vi "PID_2Chan_V4_1loop_multiTs_globals.vi"() -> ()   [LabVIEW 2016]
uses:
  <vilib>/addons/control/pid/pid.llb/PID Advanced (DBL Array).vi
  <vilib>/addons/control/pid/pid.llb/PID Parameter Manager (DBL Array).vi
  <vilib>/addons/control/pid/pid.llb/PID Derivative Action Buffered (DBL Array).vi
  <vilib>/addons/control/pid/pid.llb/PID Get Advanced Error (DBL Array).vi
  <vilib>/addons/control/pid/pid.llb/PID Integral Action Buffered (DBL Array).vi
  <vilib>/addons/control/pid/pid.llb/PID Resize 1D Array.vi
  <vilib>/addons/control/pid/pid.llb/PID Get Advanced Error (DBL).vi
  <userlib>/Fluigent/Fluigent MFCS/FluigentMFCS_Full.llb/MFCS_EZ Detect.vi
  <userlib>/Fluigent/Fluigent MFCS/FluigentMFCS_Full.llb/MFCS_EZ Initialization.vi
  <userlib>/Fluigent/Fluigent MFCS/FluigentMFCS_Full.llb/MFCS_EZ Write Channel Pressure.vi
  Globals/PressuresGlobal.vi
  <userlib>/Fluigent/Fluigent MFCS/FluigentMFCS_Full.llb/MFCS_EZ Close.vi
  <vilib>/addons/control/pid/NI_PID_pid.lvlib
  <vilib>/Analysis/NI_AALBase.lvlib
  <vilib>/Analysis/baseanly.llb/Mean (DBL).vi
panel:
  in  "Odor Mix Pressure":dbl
  in  "Set Ctr/Set Odor Mix":bool
  in  "Odor Mix Flowboard":enum16{"A", "B", "C"}(ring)
  in  "Water Mix Flowboard":enum16{"A", "B", "C"}(ring)
  in  "Ctr Water Flowboard":enum16{"A", "B", "C"}(ring)
  in  "Ctr Water":enum16{"1", "2", "3", "4", "5", "6", "7", "8"}(ring)=enum."7"
  in  "Odor Mix":enum16{"1", "2", "3", "4", "5", "6", "7", "8"}(ring)
  in  "Water Mix":enum16{"1", "2", "3", "4", "5", "6", "7", "8"}(ring)=enum."5"
  in  "Total Odor Flow":dbl=425.0
  in  "Ftot Setpoint":dbl=531.25
  in  "AutoControl PID":bool
  out "Pressure Stable?":bool=TRUE
  in  "Ftot Stability Threshold 2":dbl=0.631165
  in  "F1 Stability Threshold":dbl=0.631165
  out "Setpoint Reached?":bool
  in  "Pressure Resolution":dbl=0.631165
  in  "Control Pressure":dbl=270.0 format="%_6g"
  in  "Control Pressure Channel":i16=1
  in  "output cluster":T1
  out "Set Pressure":dbl[](array[numeric])=[924.5131355020292, 768.8474129854441] format="%_10g"
  in  "linearity":dbl[](array[numeric])=[0.30000000000000004, 0.4] format="%.2f"
  out "Flow 1 plot 2":cluster{"[0]":dbl, "[1]":dbl}(graph)={"[0]"=531.25, "[1]"=683.6630748754509}
  out "Flow Rates":dbl[](array[numeric])=[-432.47356854362795, 683.6630748754509]
  in  "FTot PID gains":cluster{"P":dbl, "I":dbl, "D":dbl}={"P"=0.02, "I"=0.0, "D"=0.0} {"D" format="%.3f"; "I" format="%.3f"; "P" format="%.5f"}
  in  "Vals to display":dbl=1235.0
  out "Flow 1 plot":cluster{"[0]":dbl, "[1]":dbl}(graph)={"[0]"=-432.47356854362795, "[1]"=225.0}
  out "Ferr":T2(graph)={"output[0]"=0.5012669198666482, "output[1]"=-3.4973900073056177, "output[2]"=0.0}
  out "Pressures":dbl[](array[numeric])=[901.3263549804688, 1487.6934814453125]
  in  "F1 PID gains":cluster{"P":dbl, "I":dbl, "D":dbl}={"P"=0.004, "I"=0.0, "D"=0.0} {"D" format="%.3f"; "I" format="%.3f"; "P" format="%.5f"}
  in  "reset Averging":bool
  in  "Set current Pressure\n to manual pressure":bool=TRUE
  out "Pressures":T3(graph)={"[0]"=901.3263549804688, "[1]"=1487.6934814453125, "[2]"=924.5131355020292, "[3]"=768.8474129854441}
  in  "stop":bool=TRUE
  in  "Control Valves":enum16{"1", "2", "3", "4", "5", "6", "7", "8"}[](array[ring])=[enum."7"]
  in  "Pressure Channels":i16[](array[numeric])=[2, 3]
  in  "reinitialize? (F)":bool
  in  "Add Ctrl?":bool
  in  "Boards":enum16{"A", "B", "C"}[](array[ring])=[enum."A", enum."A"]
  in  "Valves":enum16{"1", "2", "3", "4", "5", "6", "7", "8"}[](array[ring])=[enum."5", enum."1"]
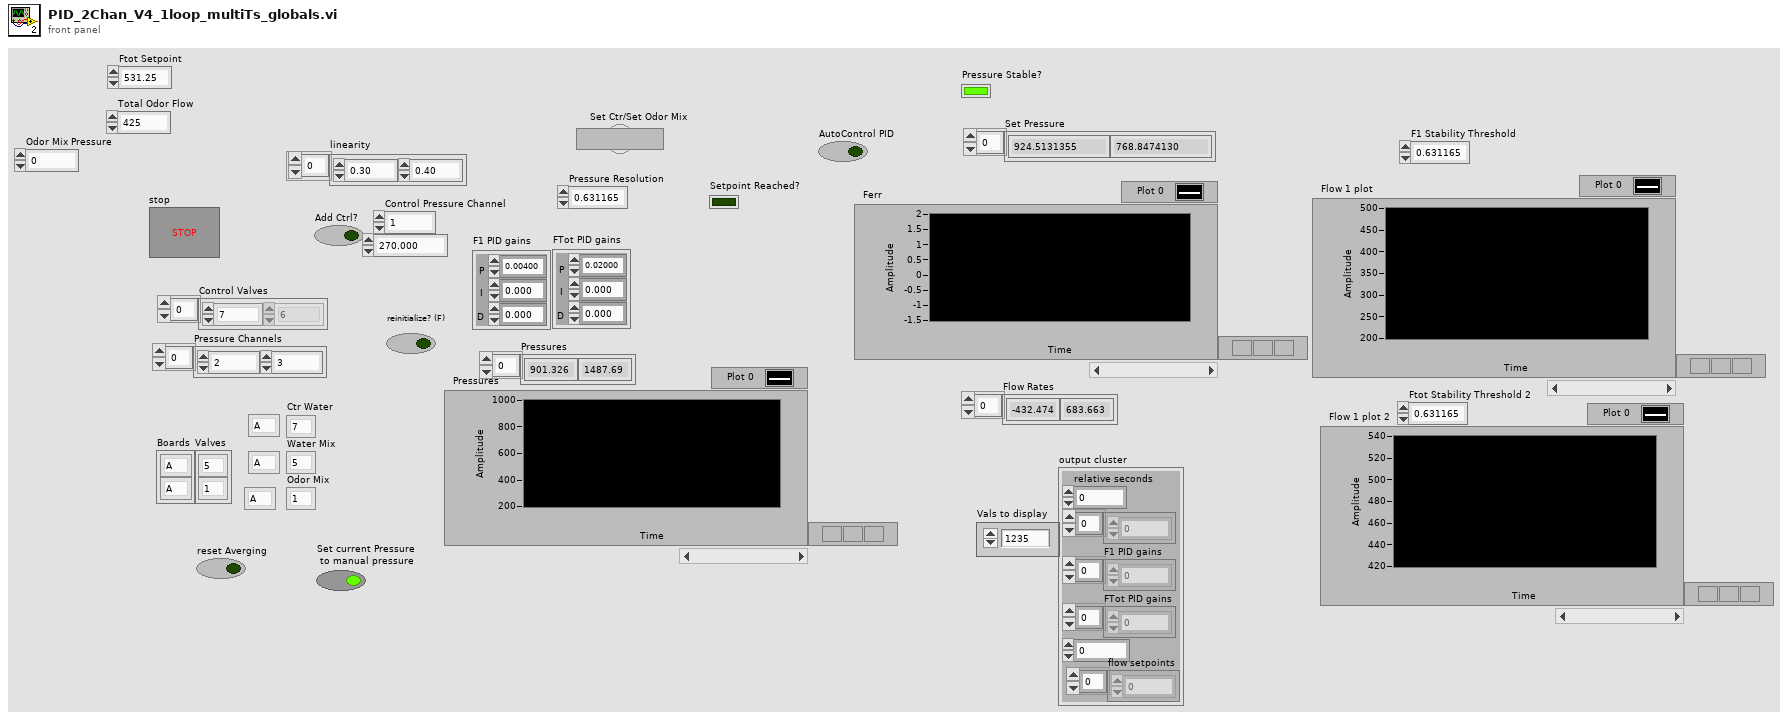
[diagram p1: front panel]
types:
  T1 = cluster{"relative seconds":dbl, "Pressures":dbl[], "F1 PID gains":dbl[], "FTot PID gains":dbl[], "PID On?":i16, "flow setpoints":dbl[]}
  T2 = cluster{"output[0]":dbl, "output[1]":dbl, "output[2]":dbl}
  T3 = cluster{"[0]":dbl, "[1]":dbl, "[2]":dbl, "[3]":dbl}
  T4 = cluster{"setpoint high":dbl, "setpoint low":dbl}[]
  T5 = typedef "_EZmfcsSN.ctl" = u16
  T6 = typedef "_EZmfcsRefNum.ctl" = refnum<k1>
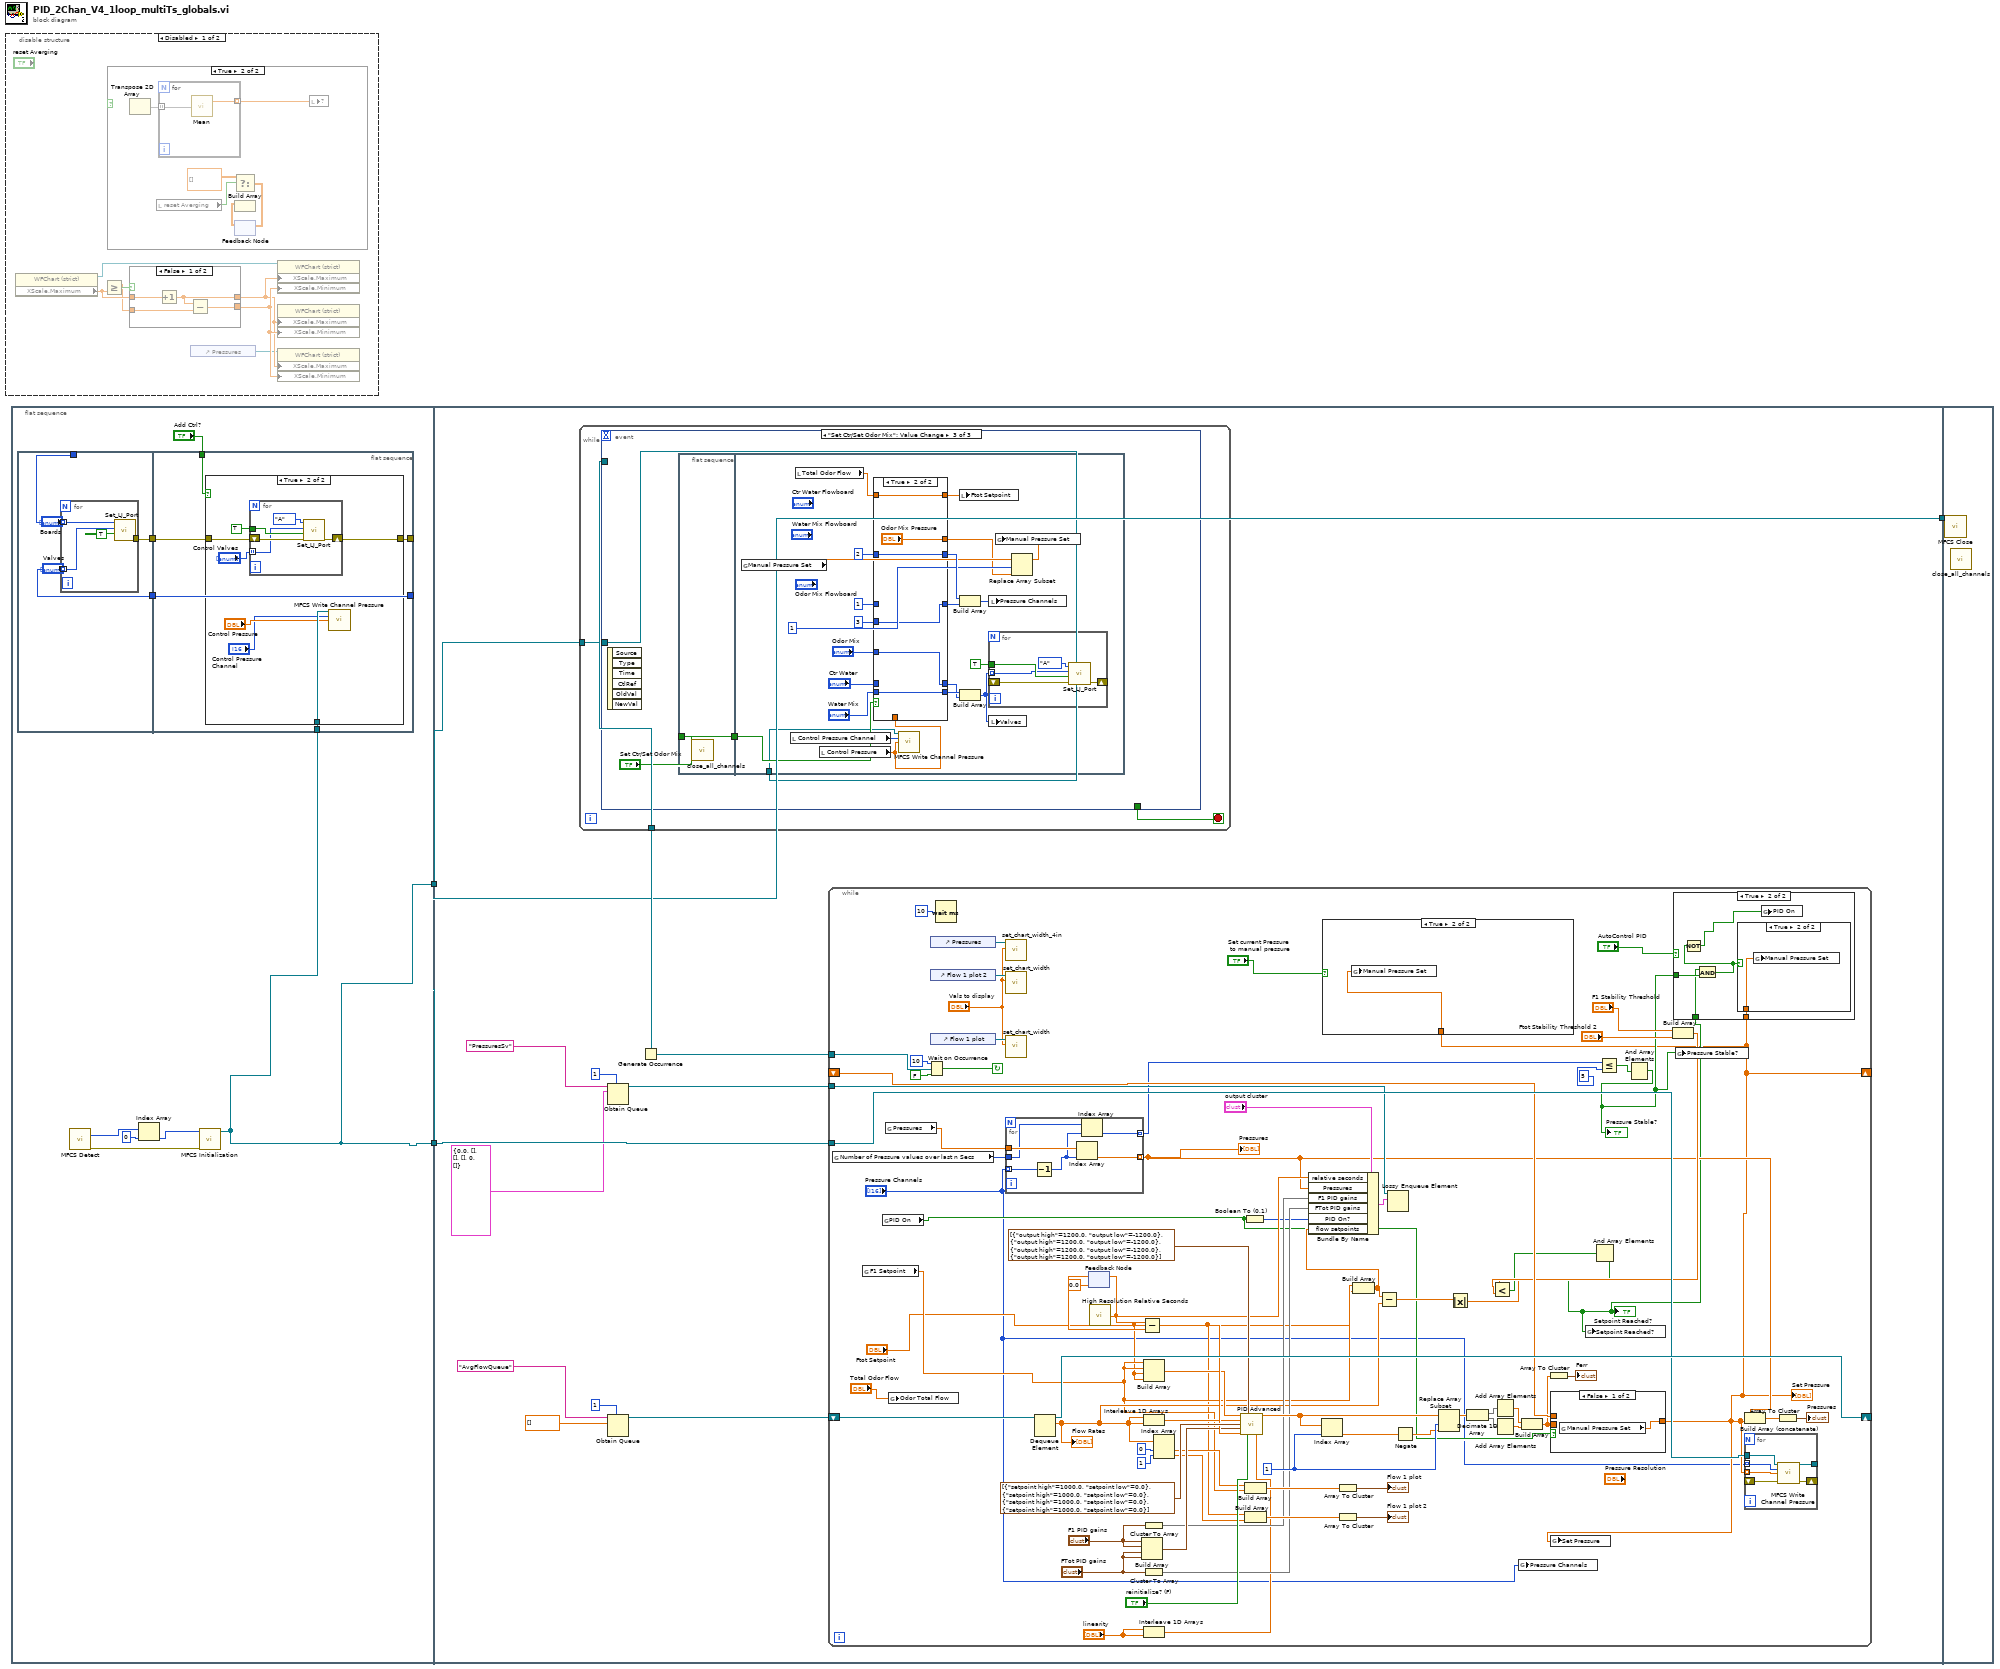
[diagram p0: block diagram]
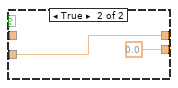
[diagram p2: hidden frame]
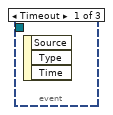
[diagram p6: hidden frame]
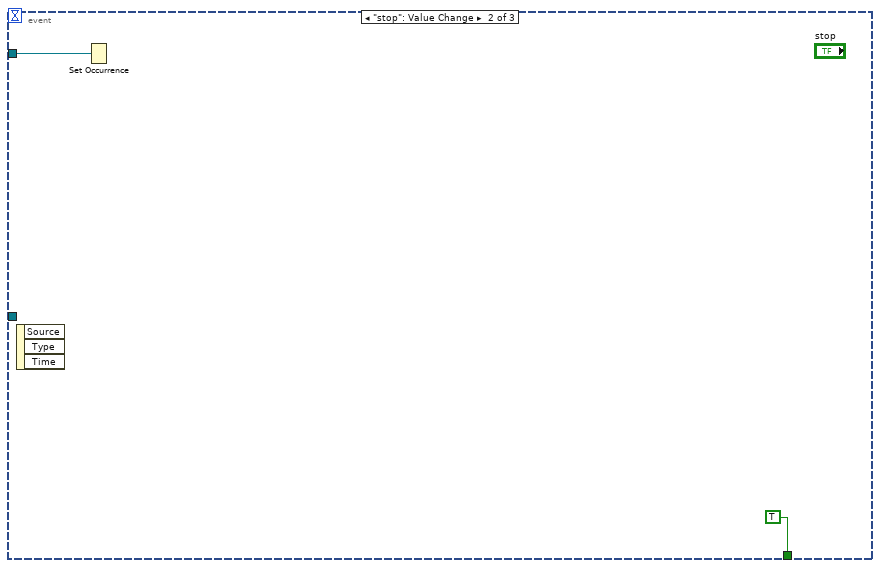
[diagram p7: hidden frame]
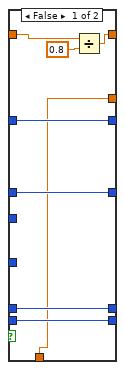
[diagram p8: hidden frame]
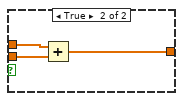
[diagram p12: hidden frame]
diagram:
  n1 = disable-structure shown="Disabled" {
    frame Disabled {
      n2 = property on="Property Node" class="WFChart (strict)"() -> (reference=w7:refnum<vi>, reference out=w8:refnum<vi>, "XScale.Maximum"=w6:dbl)  [unwired: 1 in, 1 out]
      n3 = Greater Or Equal?(y=w6) -> (x=w4:dbl, x >= y?=w5:bool)
      n4 = case shown="True" w13 {
        frame False {
        }
        frame True {
          n5 = Transpose 2D Array() -> (transposed array=w23:dbl[][])  [unwired: 1 in]
          n6 = local read "reset Averging"() -> (w24:bool)
          n7 = for {
            tunnel: w23 -> [w27] mode=indexing
            tunnel: [w26] -> w20 mode=indexing
            n8 = call-poly <vilib>:"Mean.vi"("X"=w27) -> ("mean"=w26:dbl)  [unwired: 1 out]
          }
          n9 = Select(t=dbl[][] [] ("appended array"), s=w24) -> (s? t:f=w21:dbl[][])  [unwired: 1 in]
          n10 = feedback-in #1(w21) -> ()
          n11 = feedback #1() -> (w25:dbl[][])  [unwired: 1 in]
          n12 = Build Array(w25) -> ()  [unwired: 1 in, 1 out]
          n13 = local write item#-1(w20) -> ()
        }
      }
      n14 = case shown="False" w5 {
        tunnel: w4 -> [w15 w19]
        tunnel: w6 -> [w17 _]
        tunnel: [w14 w19] -> w11
        tunnel: [w16 0.0] -> w12
        frame False {
          n15 = Increment(x=w17) -> (x+1=w14:dbl)
          n16 = Subtract(x=w14, y=w15) -> (x-y=w16:dbl)
        }
        frame True {
        }
      }
      n17 = control-ref of="Pressures"() -> (w9:refnum<vi>)
      n18 = property on="Property Node" class="WFChart (strict)"(reference=w8, "XScale.Maximum"=w11, "XScale.Minimum"=w12) -> ()  [unwired: 1 in, 2 out]
      n19 = property on="Property Node" class="WFChart (strict)"("XScale.Maximum"=w11, "XScale.Minimum"=w12) -> (reference=w10:refnum<vi>)  [unwired: 1 in, 2 out]
      n20 = property on="Property Node" class="WFChart (strict)"(reference=w9, "XScale.Maximum"=w11, "XScale.Minimum"=w12) -> ()  [unwired: 1 in, 2 out]
    }
    frame Enabled {
    }
  }
  n21 = flat-sequence {
    tunnel: [w28] -> w2
    tunnel: [w28] -> w1
    tunnel: [w63] -> w3
    tunnel: w2 -> [w63]
    tunnel: w1 -> [w61]
    tunnel: w3 -> [w224]
    frame #0 {
      n22 = flat-sequence {
        tunnel: ["Boards"] -> _
        tunnel: [w38] -> w35
        tunnel: ["Valves"] -> w34
        tunnel: [w47] -> _
        tunnel: [w45] -> _
        tunnel: w35 -> [w46]
        tunnel: w34 -> [w47]
        tunnel: "Add Ctrl?" -> [w44]
        tunnel: w28 -> [w43]
        frame #0 {
          n23 = for {
            tunnel: "Valves" -> [w42] mode=indexing
            tunnel: "Boards" -> [w41] mode=indexing
            tunnel: [w39] -> w38
            n24 = call "Set_LJ_Port.vi"("State"=TRUE, "Channel"=w42, "Flowboard"=w41) -> ("error out"=w39:errorcluster)  [unwired: 8 in]
          }
        }
        frame #1 {
          n25 = case shown="True" w44 {
            tunnel: w46 -> [w48 w55]
            tunnel: [w48 w54] -> w45
            tunnel: w43 -> [_ w51]
            frame False {
            }
            frame True {
              n26 = for {
                tunnel: TRUE ("State") -> [w58]
                shift-right: [w59] -> w54
                shift-left: w55 -> [w60]
                tunnel: "Control Valves" -> [w57] mode=indexing
                n27 = call "Set_LJ_Port.vi"("error in"=w60, "State"=w58, "Channel"=w57, "Flowboard"=enum16{"A", "B", "C"}."A") -> ("error out"=w59:errorcluster)  [unwired: 7 in]
              }
              n28 = call-poly <userlib>:"MFCS Write Channel Pressure.vi"("MFCS_EZ"=w51, "Channel Number (default=1)"="Control Pressure Channel", "Pressure (mBar)"="Control Pressure") -> ()  [unwired: 11 in, 2 out]
            }
          }
        }
      }
      n29 = call-poly <userlib>:"MFCS Detect.vi"() -> ("[SN MFCS_EZ]"=w29:T5[], "error out"=w31:errorcluster)  [unwired: 14 in]
      n30 = Index Array(array=w29, index=0) -> (element=w30:T5)
      n31 = call-poly <userlib>:"MFCS Initialization.vi"("SN MFCS_EZ"=w30, "error in (no error)"=w31) -> ("MFCS_EZ"=w28:T6)  [unwired: 11 in, 2 out]
    }
    frame #1 {
      n32 = Obtain Queue(max queue size (-1, unlimited)=1, name (unnamed)="PressuresSv", element data type=T1 {"relative seconds"=0.0, "Pressures"=[], "F1 PID gains"=[], "FTot PID gains"=[], "PID On?"=0, "flow setpoints"=[]} ("output cluster")) -> (queue out=w65:refnum<queue>)  [unwired: 2 in, 2 out]
      n33 = Obtain Queue(max queue size (-1, unlimited)=1, name (unnamed)="AvgFlowQueue", element data type=dbl[] [] ("appended array")) -> (queue out=w69:refnum<queue>)  [unwired: 2 in, 2 out]
      n34 = Generate Occurrence() -> (w68:refnum<k4>)
      n35 = while {
        tunnel: w68 -> [w74]
        tunnel: w61 -> [w73]
        stop <- w72 stop-if-true
        n36 = event shown="[2] \"Set Ctr/Set Odor Mix\": Value Change" {
          selector: _ -> [_ _ _]
          dyn-events: _ -> [_ _ _]
          timeout: _ -> [_ _ _]
          tunnel: w74 -> [_ w76 _]
          tunnel: w73 -> [_ _ w79]
          tunnel: [_ TRUE _] -> w72
          event Timeout {
            n37 = event-data() -> ()  [unwired: 1 in, 3 out]
          }
          event "stop": Value Change {
            n38 = event-data() -> ()  [unwired: 1 in, 3 out]
            n39 = Set Occurrence(w76) -> ()
          }
          event "Set Ctr/Set Odor Mix": Value Change {
            n40 = event-data() -> ()  [unwired: 1 in, 6 out]
            n41 = flat-sequence {
              tunnel: "Set Ctr/Set Odor Mix" -> [w80]
              tunnel: [w80] -> w78
              tunnel: w79 -> [w97]
              tunnel: w78 -> [w103]
              frame #0 {
                n42 = call "close_all_channels.vi"() -> ()  [unwired: 12 in]
              }
              frame #1 {
                n43 = global read "PressuresGlobal.vi" "Manual Pressure Set"() -> (w85:dbl[])
                n44 = local read "Control Pressure Channel"() -> (w98:i16)
                n45 = local read "Total Odor Flow"() -> (w87:dbl)
                n46 = local read "Control Pressure"() -> (w83:dbl)
                n47 = case shown="True" w103 {
                  tunnel: "Water Mix" -> [w114 w122]
                  tunnel: "Odor Mix" -> [_ w121]
                  tunnel: 2 -> [w116 w120]
                  tunnel: 3 -> [_ w119]
                  tunnel: [w114 w122] -> w95
                  tunnel: [w113 w121] -> w94
                  tunnel: [w116 w120] -> w92
                  tunnel: [w115 w119] -> w91
                  tunnel: 1 -> [w115 _]
                  tunnel: "Ctr Water" -> [w113 _]
                  tunnel: w87 -> [w109 w117]
                  tunnel: [w110 w117] -> w86
                  tunnel: w83 -> [w112 _]
                  tunnel: [w112 "Odor Mix Pressure"] -> w82
                  frame False {
                    n48 = Divide(x=w109, y=0.8) -> (x/y=w110:dbl)
                  }
                  frame True {
                  }
                }
                n49 = call-poly <userlib>:"MFCS Write Channel Pressure.vi"("MFCS_EZ"=w97, "Channel Number (default=1)"=w98, "Pressure (mBar)"=w83) -> ()  [unwired: 11 in, 2 out]
                n50 = local write "Ftot Setpoint"(w86) -> ()
                n51 = Build Array(w92, w91) -> (w90:i32[])
                n52 = Build Array(w95, w94) -> (w93:enum16{"1", "2", "3", "4", "5", "6", "7", "8"}[])
                n53 = local write "Pressure Channels"(w90) -> ()
                n54 = for {
                  tunnel: TRUE ("State") -> [w106]
                  shift-right: [w107] -> _
                  shift-left: _ -> [w108]
                  tunnel: w93 -> [w104] mode=indexing
                  n55 = call "Set_LJ_Port.vi"("error in"=w108, "State"=w106, "Channel"=w104, "Flowboard"=enum16{"A", "B", "C"}."A") -> ("error out"=w107:errorcluster)  [unwired: 7 in]
                }
                n56 = local write "Valves"(w93) -> ()
                n57 = Replace Array Subset(array=w85, new element=w82, index=1) -> (w81:dbl[])
                n58 = global write "PressuresGlobal.vi" "Manual Pressure Set"(w81) -> ()
              }
            }
          }
        }
      }
      n59 = while {
        shift-right: [w199] -> _
        shift-left: w69 -> [w200]
        tunnel: w68 -> [w185]
        tunnel: w63 -> [w174]
        shift-right: [w124] -> _
        shift-left: _ -> [w171]
        tunnel: w65 -> [w163]
        stop <- w184 continue-if-true
        w192 = 1 ("index")
        n60 = global read "PressuresGlobal.vi" "Number of Pressure values over last n Secs"() -> (w144:i32[])
        n61 = global read "PressuresGlobal.vi" "F1 Setpoint"() -> (w130:dbl)
        n62 = global read "PressuresGlobal.vi" "PID On"() -> (w129:bool)
        n63 = global read "PressuresGlobal.vi" "Pressures"() -> (w145:dbl[])
        n64 = global write "PressuresGlobal.vi" "Odor Total Flow"("Total Odor Flow") -> ()
        n65 = Wait on Occurrence(1:FALSE ("ignore previous (T)"), 2:w185, 3:10 ("ms timeout (-1)")) -> (0:w184:bool)
        n66 = control-ref of="Pressures"() -> (w173:refnum<vi>)
        n67 = control-ref of="Flow 1 plot 2"() -> (w157:refnum<vi>)
        n68 = control-ref of="Flow 1 plot"() -> (w156:refnum<vi>)
        n69 = Wait (ms)(milliseconds to wait=u32 10) -> ()  [unwired: 1 out]
        n70 = call "set_chart_width_4in.vi"("Values to Display"="Vals to display", "Ref In"=w173) -> ()  [unwired: 10 in]
        n71 = call "set_chart_width.vi"("Values to Display"="Vals to display", "Ctl Refnum"=w157) -> ()  [unwired: 10 in]
        n72 = call "set_chart_width.vi"("Values to Display"="Vals to display", "Ctl Refnum"=w156) -> ()  [unwired: 10 in]
        n73 = for {
          tunnel: "Pressure Channels" -> [w212] mode=indexing
          tunnel: w145 -> [w213]
          tunnel: [w211] -> w133 mode=indexing
          tunnel: w144 -> [w210]
          tunnel: [w208] -> w143 mode=indexing
          n74 = Decrement(x=w212) -> (x-1=w209:i16)
          n75 = Index Array(array=w213, index=w209) -> (element=w211:dbl)
          n76 = Index Array(array=w210, index=w209) -> (element=w208:i32)
        }
        "Pressures" <- w133
        n77 = Dequeue Element(queue=w200) -> (queue out=w199:refnum<queue>, element=w141:dbl[])  [unwired: 2 in, 2 out]
        "Flow Rates" <- w141
        n78 = feedback #2(0.0 ("relative seconds")) -> (w195:dbl)
        n79 = call <vilib>:"High Resolution Relative Seconds.vi"() -> ("relative seconds"=w162:dbl)
        n80 = feedback-in #2(w162) -> ()
        n81 = Subtract(x=w162, y=w195) -> (x-y=w194:dbl)
        n82 = Build Array("F1 PID gains", "F1 PID gains", "FTot PID gains", "FTot PID gains") -> (w188:cluster{"P":dbl, "I":dbl, "D":dbl}[])
        n83 = Build Array(w130, w130, "Ftot Setpoint", "Ftot Setpoint") -> (w182:dbl[])
        n84 = Interleave 1D Arrays(w141, w141) -> (w176:dbl[])
        n85 = Cluster To Array(cluster="F1 PID gains") -> (array=w161:dbl[])
        n86 = Cluster To Array(cluster="FTot PID gains") -> (array=w160:dbl[])
        n87 = Interleave 1D Arrays("linearity", "linearity") -> (w149:dbl[])
        n88 = Index Array(array=w141, index #1=0 ("index"), index #2=1 ("index")) -> (element #1=w154:dbl, element #2=w153:dbl)
        n89 = call-poly <vilib>:"PID Advanced.vi"("setpoint"=w182, "output range"=cluster{"output high":dbl, "output low":dbl}[] [{"output high"=1200.0, "output low"=-1200.0}, {"output high"=1200.0, "output low"=-1200.0}, {"output high"=1200.0, "output low"=-1200.0}, {"output high"=1200.0, "output low"=-1200.0}], "process variable"=w176, "setpoint range"=T4 [{"setpoint high"=1000.0, "setpoint low"=0.0}, {"setpoint high"=1000.0, "setpoint low"=0.0}, {"setpoint high"=1000.0, "setpoint low"=0.0}, {"setpoint high"=1000.0, "setpoint low"=0.0}], "PID gains"=w188, "dt (s)"=w194, "reinitialize? (F)"="reinitialize? (F)", "linearity"=w149) -> ("output"=w189:dbl[])  [unwired: 6 in, 1 out]
        n90 = Boolean To (0,1)(Boolean=w129) -> (0, 1=w159:i16)
        n91 = Build Array(w154, w130) -> (w167:dbl[])
        n92 = Build Array("Ftot Setpoint", w153) -> (w165:dbl[])
        n93 = Index Array(array=w189, index=w192) -> (element=w191:dbl)
        n94 = Array To Cluster(array=w167) -> (cluster=→"Flow 1 plot":cluster{"[0]":dbl, "[1]":dbl})
        n95 = Array To Cluster(array=w165) -> (cluster=→"Flow 1 plot 2":cluster{"[0]":dbl, "[1]":dbl})
        n96 = Build Array(w130, "Ftot Setpoint") -> (w131:dbl[])
        n97 = Bundle By Name(cluster="output cluster", "relative seconds"=w162, "Pressures"=w133, "F1 PID gains"=w161, "FTot PID gains"=w160, "PID On?"=w159, "flow setpoints"=w131) -> (w147:T1)
        n98 = Subtract(x=w131, y=w141) -> (x-y=w140:dbl[])
        n99 = Lossy Enqueue Element(queue=w163, element=w147) -> ()  [unwired: 1 in, 4 out]
        n100 = Negate(x=w191) -> (-x=w190:dbl)
        n101 = Replace Array Subset(array=w189, new element=w190, index=w192) -> (w181:dbl[])
        n102 = Absolute Value(x=w140) -> (abs(x)=w136:dbl[])
        n103 = Decimate 1D Array(w181) -> (w180:dbl[], w179:dbl[])
        n104 = Add Array Elements(numeric array=w180) -> (sum=w178:dbl)
        n105 = Add Array Elements(numeric array=w179) -> (sum=w177:dbl)
        n106 = global write "PressuresGlobal.vi" "Pressure Channels"("Pressure Channels") -> ()
        n107 = Build Array(w178, w177) -> (w170:dbl[])
        n108 = Array To Cluster(array=w170) -> (cluster=→"Ferr":cluster{"[0]":dbl, "[1]":dbl, "[2]":dbl})
        n109 = case shown="False" w129 {
          tunnel: w170 -> [_ w223]
          tunnel: w171 -> [_ w222]
          tunnel: [w220 w221] -> w124
          frame False {
            n110 = global read "PressuresGlobal.vi" "Manual Pressure Set"() -> (w220:dbl[])
          }
          frame True {
            n111 = Add(x=w222, y=w223) -> (x+y=w221:dbl[])
          }
        }
        "Set Pressure" <- w124
        n112 = case shown="True" "Set current Pressure\n to manual pressure" {
          tunnel: w124 -> [_ w207]
          frame False {
          }
          frame True {
            n113 = global write "PressuresGlobal.vi" "Manual Pressure Set"(w207) -> ()
          }
        }
        n114 = global write "PressuresGlobal.vi" "Set Pressure"(w124) -> ()
        n115 = Less Or Equal?(x=w143, y=5) -> (x <= y?=w134:bool[])
        n116 = And Array Elements(Boolean array=w134) -> (logical AND=w125:bool)
        "Pressure Stable?" <- w125
        n117 = Build Array("F1 Stability Threshold", "Ftot Stability Threshold 2") -> (w137:dbl[])
        n118 = Less?(x=w136, y=w137) -> (x < y?=w135:bool[])
        n119 = And Array Elements(Boolean array=w135) -> (logical AND=w126:bool)
        "Setpoint Reached?" <- w126
        n120 = global write "PressuresGlobal.vi" "Setpoint Reached?"(w126) -> ()
        n121 = case shown="True" "AutoControl PID" {
          tunnel: w125 -> [_ w205]
          tunnel: w126 -> [_ w204]
          tunnel: w124 -> [_ w203]
          frame False {
          }
          frame True {
            n122 = And(x=w204, y=w205) -> (x .and. y?=w202:bool)
            n123 = Not(x=w202) -> (.not. x?=w201:bool)
            n124 = case shown="True" w202 {
              tunnel: w203 -> [_ w206]
              frame False {
              }
              frame True {
                n125 = global write "PressuresGlobal.vi" "Manual Pressure Set"(w206) -> ()
              }
            }
            n126 = global write "PressuresGlobal.vi" "PID On"(w201) -> ()
          }
        }
        n127 = global write "PressuresGlobal.vi" "Pressure Stable?"(w125) -> ()
        n128 = Build Array (concatenate)(w133, w124) -> (w158:dbl[])
        n129 = for {
          shift-right: [w218] -> _
          shift-left: _ -> [w219]
          tunnel: [w217] -> _
          tunnel: "Pressure Channels" -> [w216] mode=indexing
          tunnel: w124 -> [w215] mode=indexing
          tunnel: w174 -> [w214]
          n130 = call-poly <userlib>:"MFCS Write Channel Pressure.vi"("MFCS_EZ"=w214, "Channel Number (default=1)"=w216, "Pressure (mBar)"=w215, "error in (no error)"=w219) -> ("MFCS_EZ out"=w217:T6, "error out"=w218:errorcluster)  [unwired: 10 in]
        }
        n131 = Array To Cluster(array=w158) -> (cluster=→"Pressures":T3)
      }
    }
    frame #2 {
      n132 = call-poly <userlib>:"MFCS Close.vi"("MFCS_EZ"=w224) -> ()  [unwired: 14 in, 1 out]
      n133 = call "close_all_channels.vi"() -> ()  [unwired: 12 in]
    }
  }
